vi "Enable HTTPS.vi"(7 "Private Key Password (None)":string, 8 "error in (no error)":errorcluster, 10 "HTTPS Options":T1={"HTTPS Enabled"=FALSE, "Private Key"=path "", "Private Key Format"=enum."PKCS#8 (PEM)", "Public Cert"=path "", "Public Cert Format"=enum."X.509 (PEM)", "Always Secure?"=TRUE, "HTTPS Port (443)"=433}, 11 "Server in":refnum<class "Server.lvclass">) -> (0 "error out":errorcluster, 3 "Server out":refnum<class "Server.lvclass">)   [LabVIEW 2020, in "HTTP Server.lvlib" / "Server.lvclass"]
uses:
  Server.lvclass
  HTTPS Options.ctl
  Server.lvclass/Server.ctl
  HTTP Server.lvlib
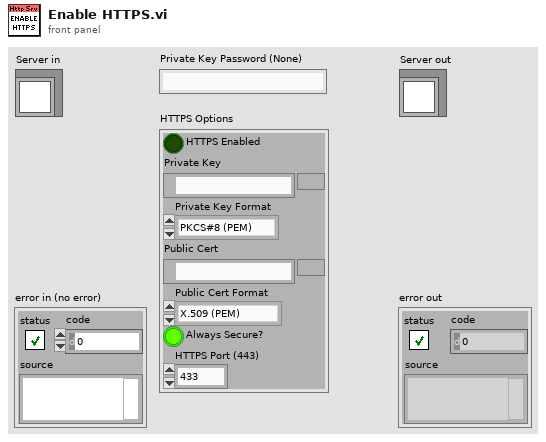
[diagram p1: front panel]
types:
  T1 = typedef "HTTP Server.lvlib/HTTPS Options.ctl" = cluster{"HTTPS Enabled":bool, "Private Key":path, "Private Key Format":enum32{"PKCS#8 (PEM)", "PKCS#8 (DER)"}, "Public Cert":path, "Public Cert Format":enum32{"X.509 (PEM)"}, "Always Secure?":bool, "HTTPS Port (443)":u16}
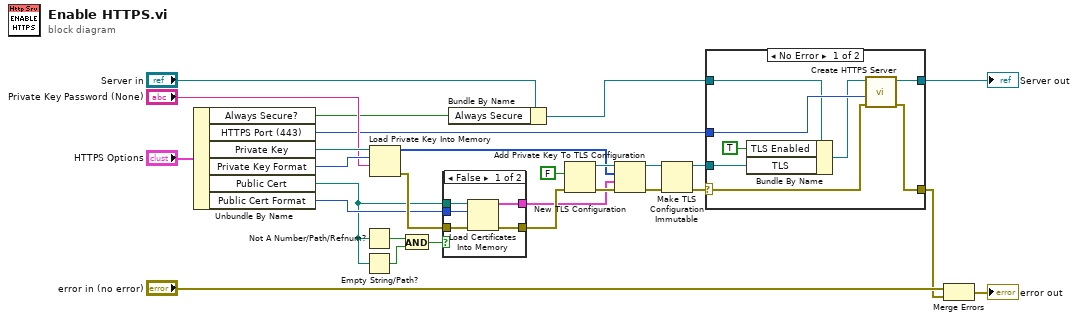
[diagram p0: block diagram]
diagram:
  n1 = Unbundle By Name("HTTPS Options") -> ("Always Secure?"=w5:bool, "HTTPS Port (443)"=w7:u16, "Private Key"=w24:path, "Private Key Format"=w23:enum32{"PKCS#8 (PEM)", "PKCS#8 (DER)"}, "Public Cert"=w4:path, "Public Cert Format"=w18:enum32{"X.509 (PEM)"})
  n2 = Not A Number/Path/Refnum?(number/path/refnum=w4) -> (NaN/Path/Refnum?=w3:bool)
  n3 = Empty String/Path?(string/path=w4) -> (empty?=w2:bool)
  n4 = Load Private Key Into Memory(9:"Private Key Password (None)", 10:w23, 11:w24) -> (0:w28:errorcluster, 3:w19:u8[])  [unwired: 1 in]
  n5 = And(x=w3, y=w2) -> (x .and. y?=w1:bool)
  n6 = case shown="False" w1 {
    tunnel: w28 -> [w33 w34]
    tunnel: [w32 w34] -> w27
    tunnel: w18 -> [w31 _]
    tunnel: [w30 _] -> w17
    tunnel: w4 -> [w29 _]
    frame False {
      n7 = Load Certificates Into Memory(8:w33, 10:w31, 11:w29) -> (0:w32:errorcluster, 3:w30:cluster{"certificate":u8[]}[])
    }
    frame True {
    }
  }
  n8 = Bundle By Name(cluster="Server in", "Always Secure"=w5) -> (w6:refnum<class "Server.lvclass">)
  n9 = New TLS Configuration(8:w27, 10:FALSE ("load OS trusted CAs?")) -> (0:w20:errorcluster, 3:w21:refnum<k36>)
  n10 = Add Private Key To TLS Configuration(8:w20, 9:w17, 10:w19, 11:w21) -> (0:w15:errorcluster, 3:w16:refnum<k36>)
  n11 = Make TLS Configuration Immutable(8:w15, 11:w16) -> (0:w14:errorcluster, 3:w12:refnum<k36>)
  n12 = case shown="No Error" w14 {
    selector: w14 -> [w40 w44]
    tunnel: w6 -> [w36 w43]
    tunnel: w12 -> [w42 _]
    tunnel: [w41 w43] -> w11
    tunnel: [w39 w44] -> w8
    tunnel: w7 -> [w38 _]
    frame No Error {
      n13 = Bundle By Name(cluster=w36, "TLS Enabled"=TRUE, "TLS"=w42) -> (w37:refnum<class "Server.lvclass">)
      n14 = call "Create HTTPS Server.vi"("error in (no error)"=w40, "Port"=w38, "Server in"=w37) -> ("error out"=w39:errorcluster, "Server out"=w41:refnum<class "Server.lvclass">)  [unwired: 7 in]
    }
    frame Error {
    }
  }
  "Server out" <- w11
  n15 = Merge Errors("error in (no error)", w8) -> (→"error out":errorcluster)
